vi "InitTracker.vi"() -> ()   [LabVIEW 2011]
panel:
  out "Array":string[](array[string])
  out "RESPONSE":string=" ON\r\n"
  in  "PORT NAME":string="Inlet_Heaters"
  # "This vi is only necessary if you have not get the special serial adaptor\nthat plugs into the front panel of the tracker module"
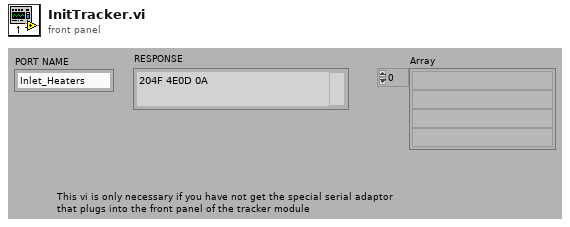
[diagram p1: front panel]
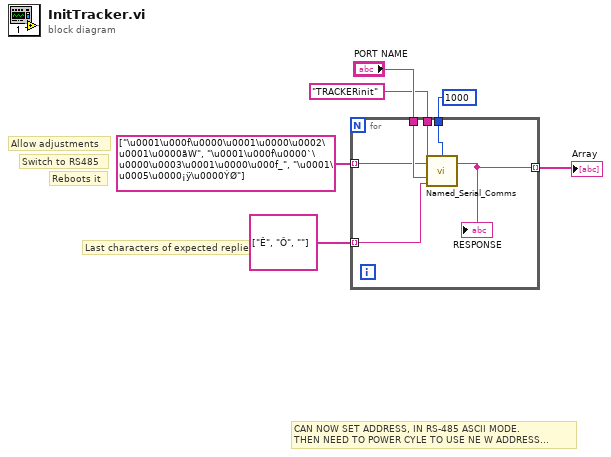
[diagram p0: block diagram]
diagram:
  # "Last characters of expected replies"
  # "CAN NOW SET ADDRESS, IN RS-485 ASCII MODE.\nTHEN NEED TO POWER CYLE TO USE NE W ADDRESS..."
  # "Switch to RS485"
  # "Allow adjustments"
  # "Reboots it"
  n1 = for {
    tunnel: "PORT NAME" -> [w12]
    tunnel: "TRACKERinit" ("Channel Name") -> [w11]
    tunnel: u32 1000 ("Timeout/ms") -> [w10]
    tunnel: string[] ["\u0001\u000f\u0000\u0001\u0000\u0002\u0001\u0000ãW", "\u0001\u000f\u0000`\u0000\u0003\u0001\u0000\u000f_", "\u0001\u0005\u0000¡ÿ\u0000ÝØ"] -> [w9] mode=indexing
    tunnel: string[] ["Ê", "Ô", ""] -> [w8] mode=indexing
    tunnel: [w7] -> w1 mode=indexing
    n2 = call "Named_Serial_Comms.vi"("Channel Name"=w11, "Write String"=w9, "Timeout/ms"=w10, "Port Name"=w12, "Term Grep"=w8) -> ("Read"=w7:string)  [unwired: 7 in, 3 out]
    "RESPONSE" <- w7
  }
  "Array" <- w1
